vi "Demo-Latest_Folder.vi"() -> ()   [LabVIEW 2020]
uses:
  <vilib>/Utility/miscctls.llb/LVRectTypeDef.ctl
  <vilib>/UPVI/lvhdf5/group.llb/H5G_obj_t.ctl
  <vilib>/UPVI/lvhdf5/file.llb/LVH5F Operation.ctl
  <vilib>/UPVI/lvhdf5/dataset.llb/LVH5D Operation.ctl
  <vilib>/Analysis/5stat.llb/RMS (DBL).vi
  <vilib>/UPVI/lvhdf5/file.llb/H5Fopen.vi
  <vilib>/UPVI/lvhdf5/utility.llb/Select HDF5 Dialog.vi
  <vilib>/UPVI/lvhdf5/utility.llb/Select HDF5 Dialog (File and Object).vi
  <vilib>/UPVI/lvhdf5/dataset.llb/Simple H5Dread (Variant).vi
  <vilib>/UPVI/lvhdf5/utility.llb/Select HDF5 Dialog (Object Only).vi
  <vilib>/UPVI/lvhdf5/dataset.llb/Simple H5Dread.xnode
  <vilib>/UPVI/lvhdf5/library.llb/HDF5 Ref.ctl
  <vilib>/UPVI/lvhdf5/library.llb/HDF5 Ref.lvclass
  <vilib>/UPVI/lvhdf5/file.llb/H5Fclose.vi
  <vilib>/UPVI/lvhdf5/identifier.llb/Not an HDF5 Refnum Constant.vi
  <vilib>/UPVI/lvhdf5/dataset.llb/OpenCreateReplace Dataset.vi
  <vilib>/UPVI/lvhdf5/dataset.llb/H5Dget_space.vi
  <vilib>/UPVI/lvhdf5/dataspace.llb/H5Sget_simple_extent_dims.vi
  <vilib>/UPVI/lvhdf5/dataspace.llb/H5Sselect_hyperslab.vi
  <vilib>/UPVI/lvhdf5/dataset.llb/H5Dread (Variant).vi
  <vilib>/UPVI/lvhdf5/attribute.llb/private/LVH5AreadWDTAttrs.vi
  <vilib>/UPVI/lvhdf5/dataspace.llb/H5Sclose.vi
  <vilib>/Utility/error.llb/Error Cluster From Error Code.vi
  <vilib>/UPVI/lvhdf5/dataset.llb/H5Dclose.vi
  <vilib>/Analysis/NI_AALBase.lvlib
  <vilib>/Analysis/NI_AALPro.lvlib
panel:
  out "Standard Deviation div. Mean":dbl
  out "rms value":dbl format="%0.2f"
  out "variance":dbl format="%0.2f"
  out "standard deviation":dbl format="%0.2f"
  out "mean":dbl format="%0.2f"
  out "Metrics Histogram":T1(graph)
  in  "Stop":bool
  out "HDF5 file path":path
  in  "Folder to Monitor":path=path "T:/2022-07-19"
  in  "Basename":string="Net15 Nucleo H7 Photodiode"
  out "Metrics Temporal Plot":cluster{u64[], "Data out":dbl[]}(graph)
  # "Simple Demo of Metrics Visualization from an Existing HDF5 File"
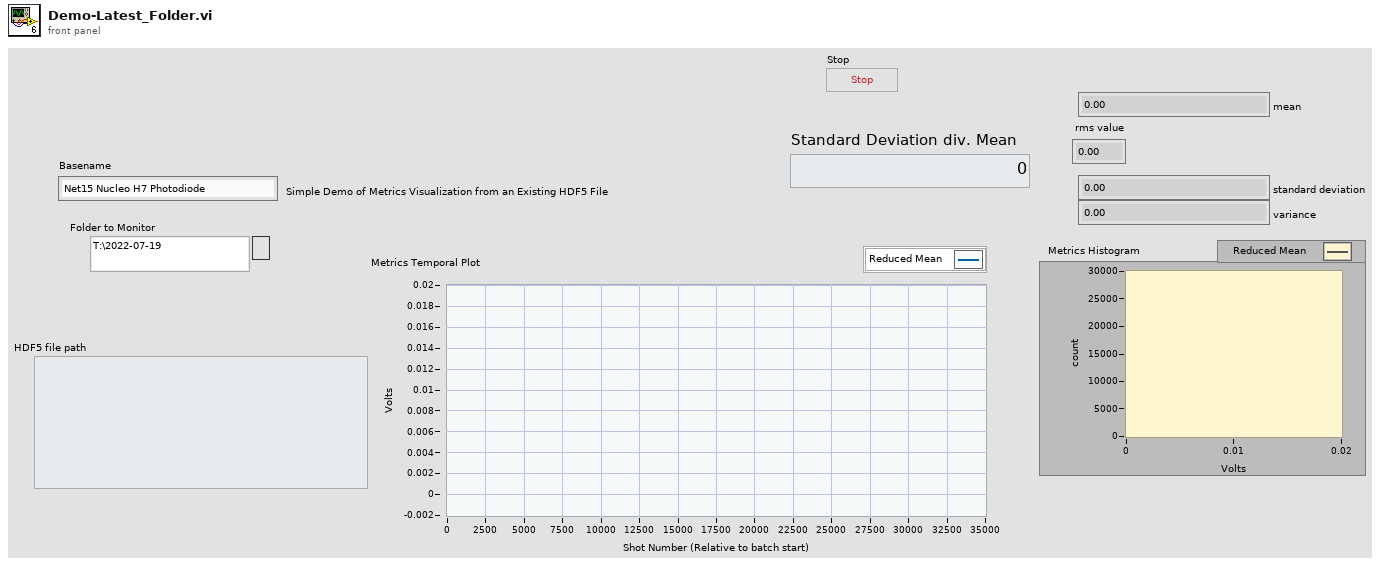
[diagram p1: front panel]
types:
  T1 = cluster{"X Values":dbl[], "Histogram: h(x)":i32[]}
  T2 = typedef "LVRectTypeDef.ctl" = cluster{"Left":i16, "Top":i16, "Right":i16, "Bottom":i16}
  T3 = cluster{"Behavior":enum32{"Invalid", "Default", "Floating", "Floating/Auto-Hide", "Modal"}, "Position":T2, "Center":bool, "Title":string}
  T4 = typedef "LVH5D Operation.ctl" = enum16{"open", "replace", "create", "open or create", "create or replace", "create or replace with confirmation"}
  T5 = typedef "LVH5F Operation.ctl" = enum16{"open", "open or create", "create or replace", "create or replace (with confirmation)", "create", "open (read only)"}
  T6 = typedef "H5G_obj_t.ctl" = i32
  T7 = cluster{"Object Types (any)":T6[], "Object Pattern":string}
  T8 = typedef "HDF5 Ref.ctl" = refnum<class "HDF5 Ref.lvclass">
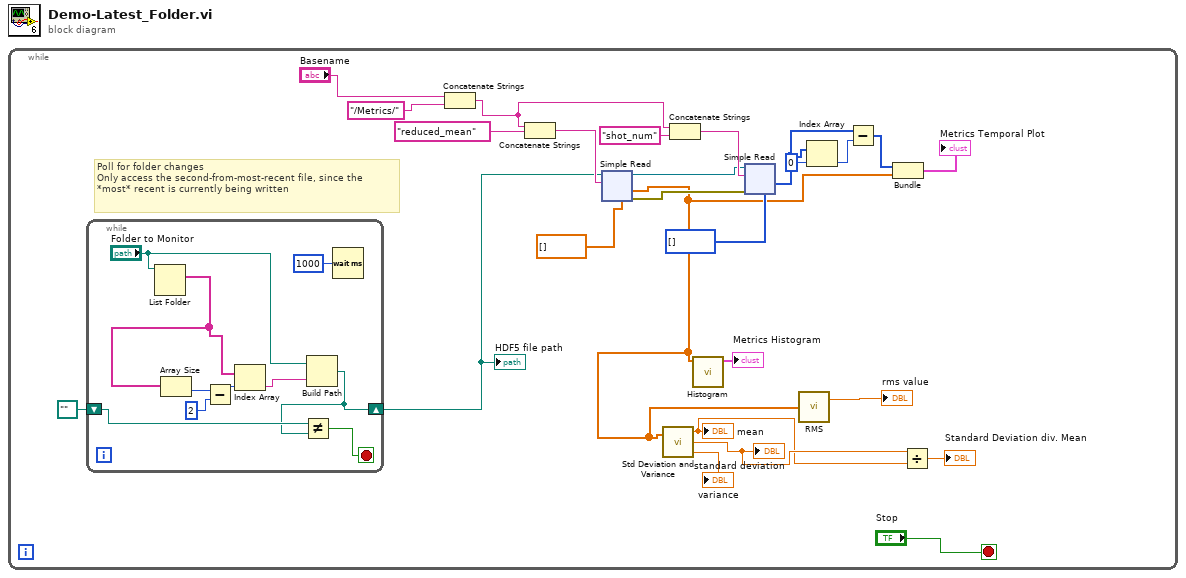
[diagram p0: block diagram]
diagram:
  n1 = while {
    stop <- "Stop" stop-if-true
    # "Poll for folder changes\nOnly access the second-from-most-recent file, since the *most* recent is currently being written"
    n2 = while {
      shift-right: [w30] -> w13
      shift-left: path "" ("appended path") -> [w34]
      stop <- w33 stop-if-true
      n3 = List Folder(path="Folder to Monitor") -> (filenames=w36:string[])  [unwired: 3 in, 3 out]
      n4 = Array Size(array=w36) -> (size(s)=w28:i32)
      n5 = Subtract(x=w28, y=2) -> (x-y=w29:i32)
      n6 = Index Array(array=w36, index=w29) -> (element=w35:string)
      n7 = Build Path(base path="Folder to Monitor", name or relative path=w35) -> (appended path=w30:path)
      n8 = Not Equal?(x=w34, y=w30) -> (x != y?=w33:bool)
      n9 = Wait (ms)(milliseconds to wait=u32 1000) -> ()  [unwired: 1 out]
    }
    "HDF5 file path" <- w13
    n10 = Concatenate Strings("Basename", "/Metrics/") -> (w10:string)
    n11 = Concatenate Strings(w10, "reduced_mean" ("Dataset Path")) -> (w24:string)
    n12 = xnode "Simple Read"("Dataset Path"=w24, "HDF5 Path or Ref"=w13, "Data"=dbl[] []) -> ("HDF5 Ref out"=w21:T8, "error out"=w18:errorcluster, "Data out"=w5:dbl[])  [unwired: 1 in, 1 out]
    n13 = call <vilib>:"Std Deviation and Variance.vi"("X"=w5) -> ("mean"=w2:dbl, "standard deviation"=w3:dbl, "variance"=→"variance":dbl)  [unwired: 1 in]
    "mean" <- w2
    "standard deviation" <- w3
    n14 = Concatenate Strings(w10, "shot_num" ("string")) -> (w22:string)
    n15 = call <vilib>:"Histogram.vi"("X"=w5) -> ("Histogram Graph"=→"Metrics Histogram":T1)  [unwired: 7 in, 3 out]
    n16 = xnode "Simple Read"("Dataset Path"=w22, "error in (no error)"=w18, "HDF5 Path or Ref"=w21, "Data"=u64[] []) -> ("Data out"=w15:u64[])  [unwired: 3 out]
    n17 = call-poly <vilib>:"RMS.vi"("X"=w5) -> ("rms value"=→"rms value":dbl)  [unwired: 1 out]
    n18 = Index Array(array=w15, index=0) -> (element=w16:u64)
    n19 = Subtract(x=w15, y=w16) -> (x-y=w14:u64[])
    n20 = Bundle(w14, "Data out"=w5) -> (→"Metrics Temporal Plot":cluster{u64[], "Data out":dbl[]})  [unwired: 1 in]
    n21 = Divide(x=w3, y=w2) -> (x/y=→"Standard Deviation div. Mean":dbl)
  }
